vi "Act2_BaseDatos_IV.vi"() -> ()   [LabVIEW 2020]
uses:
  <vilib>/httpClient/PUTBuffer.vi
  <vilib>/httpClient/LabVIEWHTTPClient.lvlib
panel:
  out "body PUT":string
  out "headers PUT":string
  in  "Fecha":string
  in  "Horizontal Pointer Slider":dbl(slide) scale=0.0..10.0
  in  "Vertical Pointer Slider":dbl(slide) scale=0.0..10.0
  in  "Lateral":bool
  in  "Frontal":bool
  out "error PUT":errorcluster
  out "error out":errorcluster
  in  "stop":bool
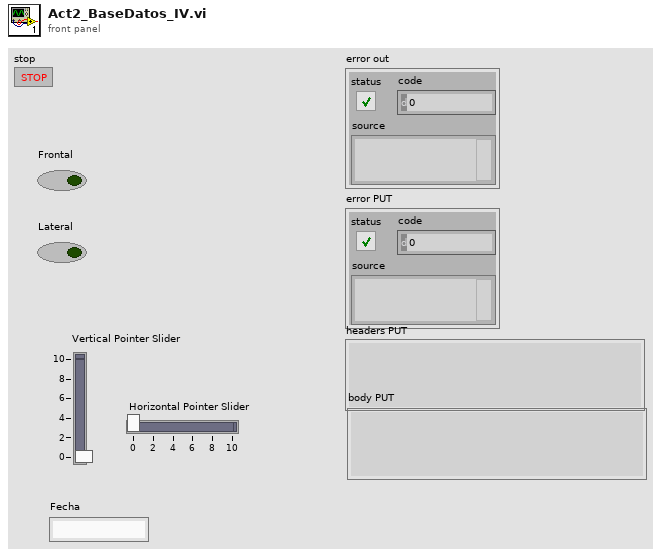
[diagram p1: front panel]
types:
  T1 = cluster{"Fecha":string, "Humedad":dbl, "Temperatura":dbl}
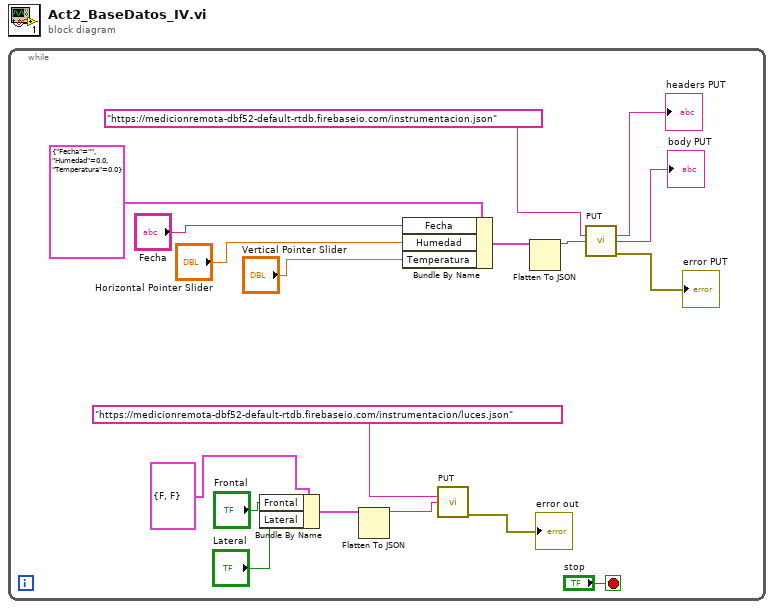
[diagram p0: block diagram]
diagram:
  n1 = while {
    stop <- "stop" stop-if-true
    n2 = Bundle By Name(cluster=cluster{"Lateral":bool, "Frontal":bool} {"Lateral"=FALSE, "Frontal"=FALSE}, "Frontal"="Frontal", "Lateral"="Lateral") -> (w15:cluster{"Lateral":bool, "Frontal":bool})
    n3 = Flatten To JSON(anything=w15) -> (JSON string=w3:string)  [unwired: 2 in, 1 out]
    n4 = Bundle By Name(cluster=T1 {"Fecha"="", "Humedad"=0.0, "Temperatura"=0.0}, "Fecha"="Fecha", "Humedad"="Horizontal Pointer Slider", "Temperatura"="Vertical Pointer Slider") -> (w9:T1)
    n5 = call-poly <vilib>:"PUT.vi"("url"="https://medicionremota-dbf52-default-rtdb.firebaseio.com/instrumentacion/luces.json", "buffer"=w3) -> ("error out"=→"error out":errorcluster)  [unwired: 10 in, 3 out]
    n6 = Flatten To JSON(anything=w9) -> (JSON string=w8:string)  [unwired: 2 in, 1 out]
    n7 = call-poly <vilib>:"PUT.vi"("url"="https://medicionremota-dbf52-default-rtdb.firebaseio.com/instrumentacion.json", "buffer"=w8) -> ("headers"=→"headers PUT":string, "body"=→"body PUT":string, "error out"=→"error PUT":errorcluster)  [unwired: 10 in, 1 out]
  }
